vi "Init.vi"(7 "Prepend Result Name":bool, 8 "error in (no error)":errorcluster, 9 "DC Pins":string[](array[string]), 10 "Measurement Name":string) -> (0 "error out":errorcluster, 3 "DCLeakage out":refnum<class "DCLeakage.lvclass">)   [LabVIEW 2018, in "SeqAuto Evaluations.lvlib" / "DCLeakage.lvclass"]
uses:
  DCLeakage.lvclass
  C:/Sequence Automation/Plugins/SeqAuto IEvaluation.lvlibp/SeqAuto IEvaluation.lvclass
  DCLeakage.lvclass/DCLeakage.ctl
  Write DC Pins.vi
  Plugins/SeqAuto IEvaluation.lvlibp/Write Measurement Name.vi
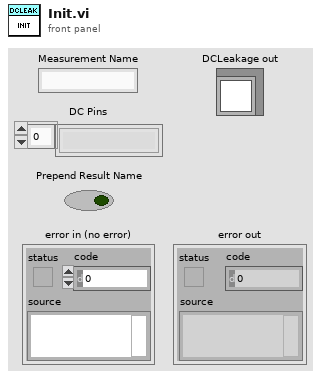
[diagram p1: front panel]
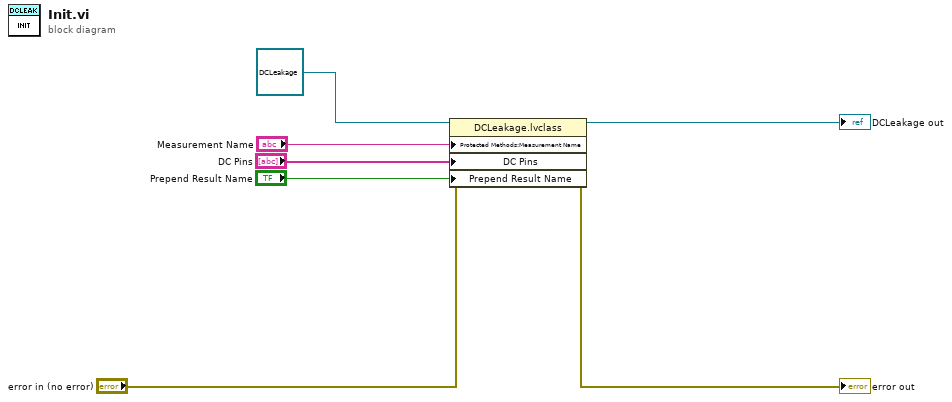
[diagram p0: block diagram]
diagram:
  n1 = property class="DCLeakage.lvclass"(reference=refnum<class "DCLeakage.lvclass"> refnum ("DCLeakage in"), error in="error in (no error)", "Protected Methods:Measurement Name"="Measurement Name", "DC Pins"="DC Pins", "Prepend Result Name"="Prepend Result Name") -> (reference out=→"DCLeakage out":refnum<class "DCLeakage.lvclass">, error out=→"error out":errorcluster)
